vi "Adjust Idle Benchmark.vi"(11 "CIFCorePlugin in":refnum<class "CIFCorePlugin.lvclass">) -> (3 "CIFCorePlugin out":refnum<class "CIFCorePlugin.lvclass">)   [LabVIEW 2021, in "CIFCorePlugin.lvclass"]
uses:
  CIFCorePlugin.lvclass
  CIFCorePlugin.lvclass/CIFCorePlugin.ctl
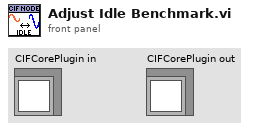
[diagram p1: front panel]
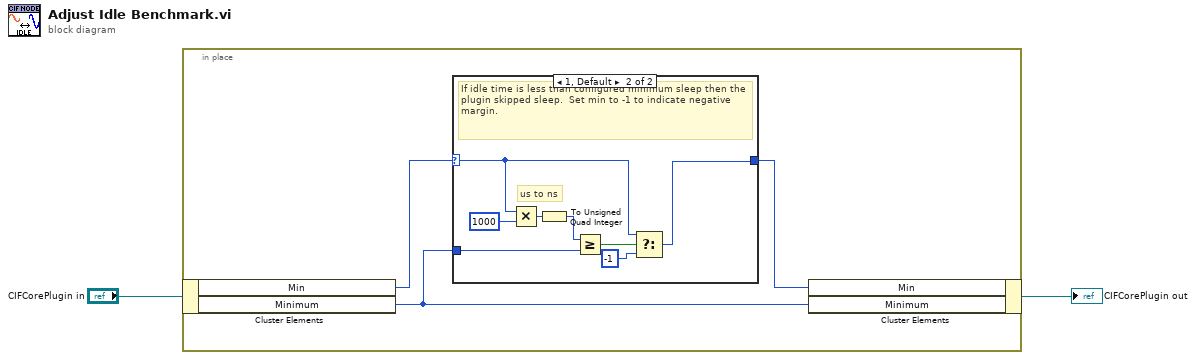
[diagram p0: block diagram]
diagram:
  n1 = in-place {
    n2 = in-place-cluster #1("CIFCorePlugin in") -> ("Min"=w3:i32, "Minimum"=w5:u64)
    n3 = case shown="1, Default" w3 {
      selector: w3 -> [w6 w9]
      tunnel: w5 -> [_ w14]
      tunnel: [w6 w11] -> w4
      frame 0 {
        # "Default value"
      }
      frame 1, Default {
        # "us to ns"
        # "If idle time is less than configured minimum sleep then the plugin skipped sleep.  Set min to -1 to indicate negative margin."
        n4 = Multiply(x=w9, y=1000) -> (x*y=w8:i32)
        n5 = To Unsigned Quad Integer(1:w8) -> (0:w13:u64)
        n6 = Greater Or Equal?(x=w13, y=w14) -> (x >= y?=w12:bool)
        n7 = Select(t=w9, s=w12, f=-1) -> (s? t:f=w11:i32)
      }
    }
    n8 = in-place-cluster #1("Min"=w4, "Minimum"=w5) -> (→"CIFCorePlugin out":refnum<class "CIFCorePlugin.lvclass">)
  }
